vi "DeviceToDigitalOutput.vi"(8 "error in (no error)":errorcluster, 11 "TesteractHAL_Device In":refnum<class "TesteractHAL_Device.lvclass">) -> (0 "error out":errorcluster, 3 "TesteractHAL_DigitalIO Out":refnum<class "TesteractHAL_DigitalOutput.lvclass">)   [LabVIEW 2017, in "TesteractHAL_DigitalOutput.lvlib" / "TesteractHAL_DigitalOutput.lvclass"]
doc: "Converts the Device object into a DigitalIO object.\n\nIgnores errors and just passes them through."
uses:
  TesteractHAL_DigitalOutput.lvclass
  Program Files (x86)/Testeract/HWLib/HAL/Device/TesteractHAL_Device.lvlibp/TesteractHAL_Device.lvclass
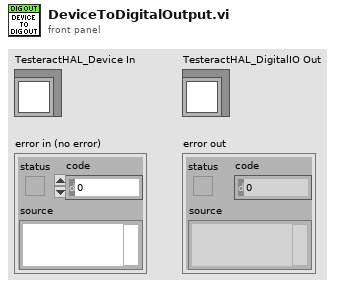
[diagram p1: front panel]
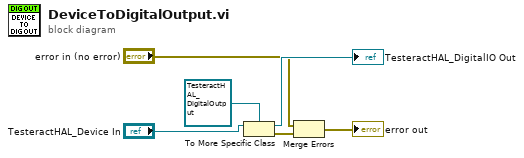
[diagram p0: block diagram]
diagram:
  n1 = To More Specific Class(target class=refnum<class "TesteractHAL_DigitalOutput.lvclass"> refnum ("DigitalIO.lvlib:DigitalIO.lvclass"), reference="TesteractHAL_Device In") -> (specific class reference=→"TesteractHAL_DigitalIO Out":refnum<class "TesteractHAL_DigitalOutput.lvclass">, error out=w4:errorcluster)  [unwired: 1 in]
  n2 = Merge Errors("error in (no error)", w4) -> (→"error out":errorcluster)
